vi "IV 3MV5 P01 MMME.vi"(0 "Botonera":bool[](array[boolean])) -> (1 "D0":T1, 2 "D1":T1, 3 "D2":T1)   [LabVIEW 2021]
doc: "Programa que permite el cambio de 7 bits a numeros decimales observables en los displays de 7 segmentos, separándo los valores en Unidades (D2) Decenas (D1) Centenas (D0)\n- Creador: Mendoza Meza Manuel Everardo\n- Grupo: 3MV5\n- Periodo: 2022/2"
panel:
  # "Mendoza Meza Manuel Everardo"
  # "Centenas"
  # "Decenas"
  # "Unidades"
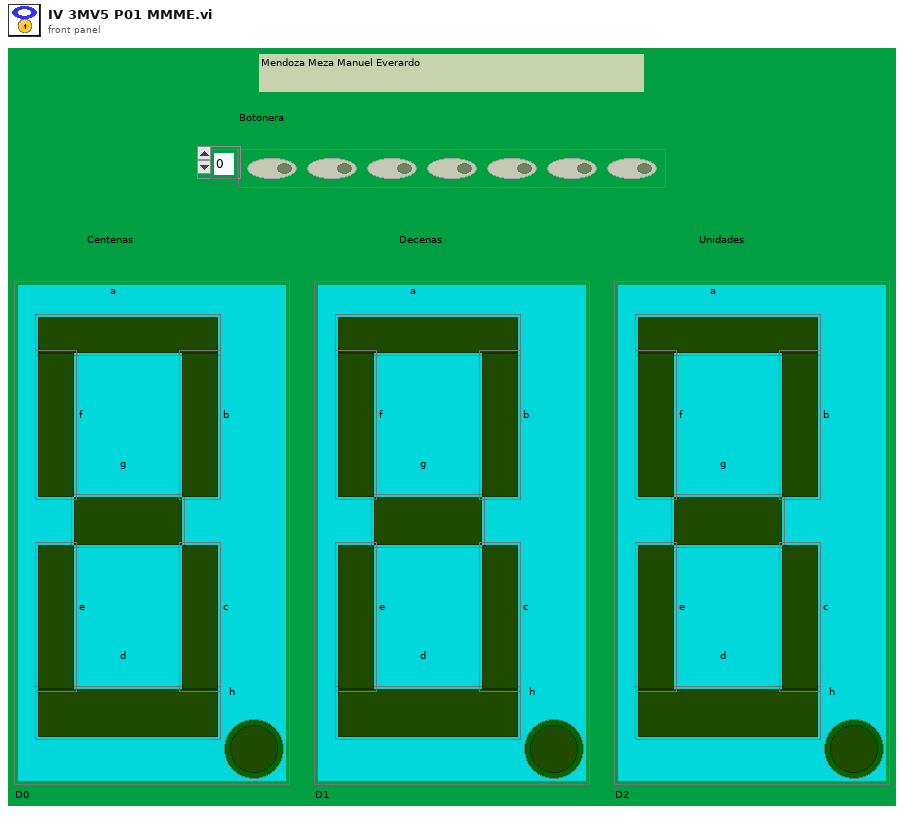
[diagram p1: front panel]
types:
  T1 = cluster{"a":bool, "g":bool, "d":bool, "b":bool, "f":bool, "c":bool, "e":bool, "h":bool}
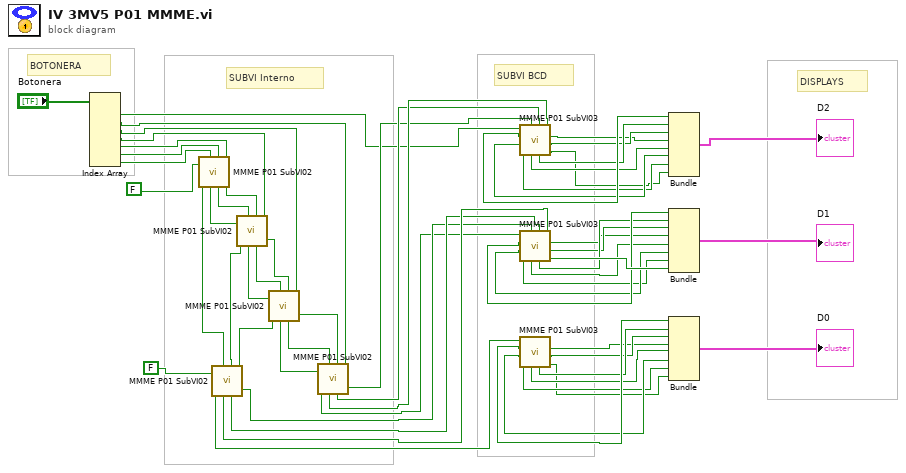
[diagram p0: block diagram]
diagram:
  # "BOTONERA"
  # "SUBVI BCD"
  # "SUBVI Interno"
  # "DISPLAYS"
  n1 = Index Array(array="Botonera") -> (element #1=w1:bool, element #2=w47:bool, element #3=w48:bool, element #4=w49:bool, element #5=w50:bool, element #6=w51:bool, element #7=w52:bool)  [unwired: 7 in]
  n2 = call "MMME P01 SubVI02.vi"("A"=FALSE, "B"=w52, "C"=w51, "D"=w50) -> ("W"=w40:bool, "X"=w56:bool, "Y"=w55:bool, "Z"=w54:bool)
  n3 = call "MMME P01 SubVI02.vi"("A"=w56, "B"=w55, "C"=w54, "D"=w49) -> ("W"=w38:bool, "X"=w46:bool, "Y"=w45:bool, "Z"=w44:bool)
  n4 = call "MMME P01 SubVI02.vi"("A"=w46, "B"=w45, "C"=w44, "D"=w48) -> ("W"=w37:bool, "X"=w43:bool, "Y"=w42:bool, "Z"=w41:bool)
  n5 = call "MMME P01 SubVI02.vi"("A"=FALSE, "B"=w40, "C"=w38, "D"=w37) -> ("W"=w36:bool, "X"=w8:bool, "Y"=w7:bool, "Z"=w6:bool)
  n6 = call "MMME P01 SubVI02.vi"("A"=w43, "B"=w42, "C"=w41, "D"=w47) -> ("W"=w5:bool, "X"=w4:bool, "Y"=w3:bool, "Z"=w2:bool)
  n7 = call "MMME P01 SubVI03.vi"("D"=w4, "C"=w3, "B"=w2, "A"=w1) -> ("h"=w28:bool, "d"=w33:bool, "b"=w32:bool, "g"=w34:bool, "f"=w31:bool, "e"=w29:bool, "c"=w30:bool, "a"=w35:bool)
  n8 = call "MMME P01 SubVI03.vi"("D"=w8, "C"=w7, "B"=w6, "A"=w5) -> ("h"=w18:bool, "d"=w15:bool, "b"=w14:bool, "g"=w16:bool, "f"=w13:bool, "e"=w11:bool, "c"=w12:bool, "a"=w17:bool)
  n9 = call "MMME P01 SubVI03.vi"("A"=w36) -> ("h"=w19:bool, "d"=w24:bool, "b"=w23:bool, "g"=w25:bool, "f"=w22:bool, "e"=w20:bool, "c"=w21:bool, "a"=w26:bool)  [unwired: 3 in]
  n10 = Bundle("a"=w35, "g"=w34, "d"=w33, "b"=w32, "f"=w31, "c"=w30, "e"=w29, "h"=w28) -> (→"D2":T1)  [unwired: 1 in]
  n11 = Bundle("a"=w17, "g"=w16, "d"=w15, "b"=w14, "f"=w13, "c"=w12, "e"=w11, "h"=w18) -> (→"D1":T1)  [unwired: 1 in]
  n12 = Bundle("a"=w26, "g"=w25, "d"=w24, "b"=w23, "f"=w22, "c"=w21, "e"=w20, "h"=w19) -> (→"D0":T1)  [unwired: 1 in]
